vi "Get one point_test.vi"() -> ()   [LabVIEW 2017]
uses:
  <vilib>/DAQmx/read.llb/DAQmx Read (Analog DBL 1Chan 1Samp).vi
  <vilib>/DAQmx/write.llb/DAQmx Write (Analog DBL 1Chan 1Samp).vi
  <vilib>/DAQmx/create/channels.llb/DAQmx Create Channel (AO-Voltage-Basic).vi
  <vilib>/DAQmx/configure/timing.llb/DAQmx Timing (Sample Clock).vi
  <vilib>/DAQmx/create/channels.llb/DAQmx Create Channel (AI-Voltage-Basic).vi
  <vilib>/DAQmx/configure/trigger.llb/DAQmx Start Trigger (Digital Edge).vi
  <vilib>/DAQmx/configure/trigger.llb/DAQmx Start Trigger (Analog Edge).vi
  <vilib>/DAQmx/miscellaneous.llb/DAQmx Fill In Error Info.vi
panel:
  out "Time 4":dbl format="%_19f"
  out "Time 3":dbl format="%_19f"
  out "Time 2":dbl format="%_19f"
  out "Time 1":dbl format="%_19f"
  out "data":dbl format="%0.2f"
  in  "Sample Rate":dbl=500000.0 format="%.3p"
  in  "Voltage Read":tag="Dev1/ai1"
  in  "Gate":tag="Dev1/ao0"
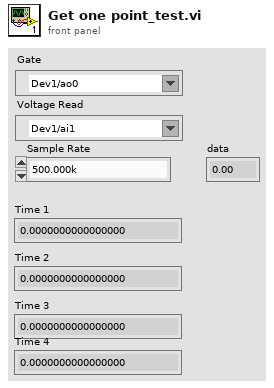
[diagram p1: front panel]
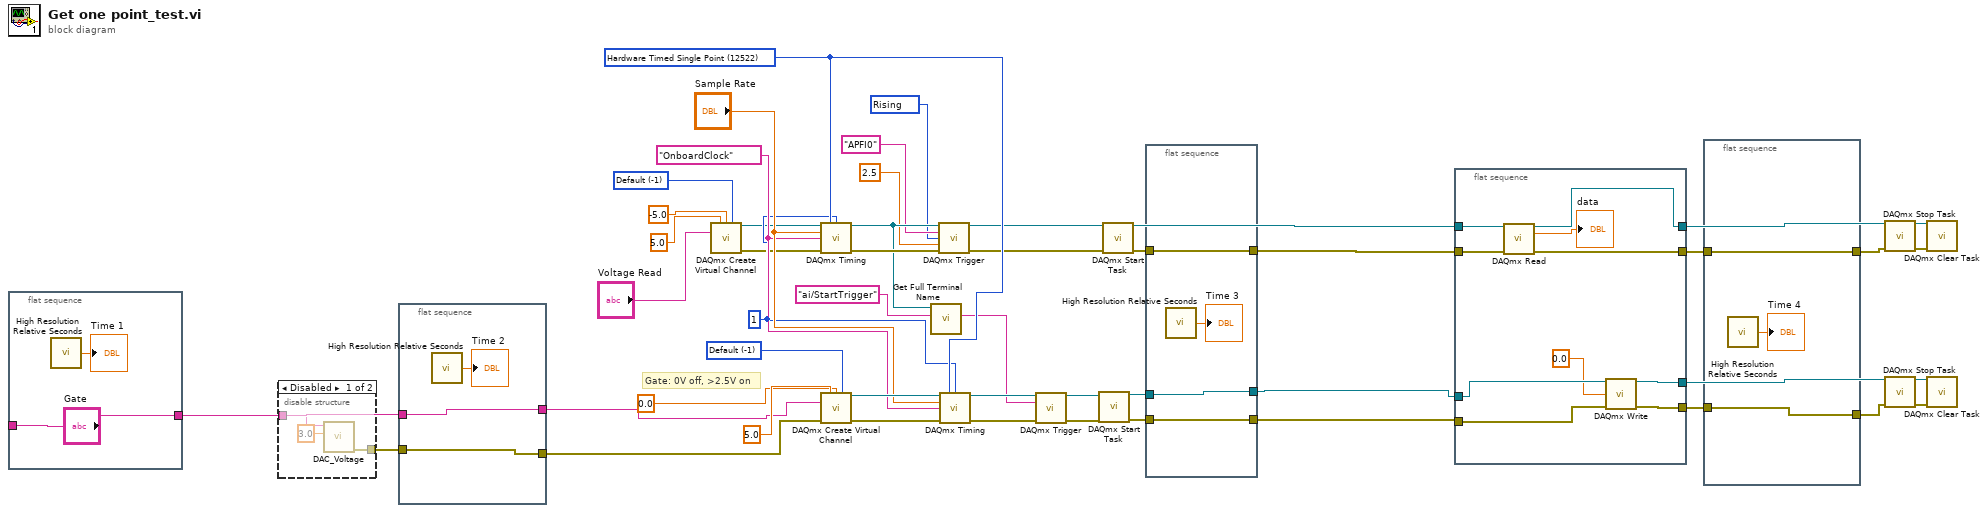
[diagram p0: block diagram]
diagram:
  w16 = 10280 items=["Rising"=10280, "Falling"=10171] ("slope")
  w36 = -1 items=["Default"=-1, "RSE"=10083, "NRSE"=10078, "Differential"=10106, "Pseudodifferential"=12529] ("input terminal configuration")
  w42 = 1 ("samples per channel")
  w43 = 12522 items=["Finite Samples"=10178, "Continuous Samples"=10123, "Hardware Timed Single Point"=12522] ("sample mode")
  w44 = tag "OnboardClock" ("source")
  w48 = -1 items=["Default"=-1, "RSE"=10083, "Differential"=10106, "Pseudodifferential"=12529] ("output terminal configuration")
  # "Gate: 0V off, >2.5V on"
  n1 = flat-sequence {
    tunnel: [w52] -> w13
    tunnel: "Gate" -> [w52]
    frame #0 {
      n2 = call <vilib>:"High Resolution Relative Seconds.vi"() -> ("relative seconds"=→"Time 1":dbl)
    }
  }
  n3 = disable-structure shown="Disabled" {
    disable-tunnel: w13 -> [w55 _]
    disable-tunnel: [w54 _] -> w11
    frame Disabled {
      n4 = call "DAC_Voltage.vi"("Voltage"=3.0, "Physical Channel(s)"=w55) -> ("error out"=w54:errorcluster)  [unwired: 9 in]
    }
    frame Enabled {
    }
  }
  n5 = flat-sequence {
    tunnel: [w58] -> w14
    tunnel: w13 -> [w58]
    tunnel: [w57] -> w12
    tunnel: w11 -> [w57]
    frame #0 {
      n6 = call <vilib>:"High Resolution Relative Seconds.vi"() -> ("relative seconds"=→"Time 2":dbl)
    }
  }
  n7 = call-poly <vilib>:"DAQmx Create Virtual Channel.vi"("maximum value"=5.0, "minimum value"=-5.0, "input terminal configuration"=w36, "physical channels"="Voltage Read") -> ("task out"=w35:refnum<k21>, "error out"=w34:errorcluster)  [unwired: 10 in]
  n8 = call-poly <vilib>:"DAQmx Timing.vi"("task/channels in"=w35, "sample mode"=w43, "samples per channel"=w42, "rate"="Sample Rate", "source"=w44, "error in"=w34) -> ("task out"=w20:refnum<k21>, "error out"=w33:errorcluster)  [unwired: 8 in]
  n9 = call-poly <vilib>:"DAQmx Create Virtual Channel.vi"("maximum value"=5.0, "minimum value"=0.0, "output terminal configuration"=w48, "physical channels"=w14, "error in"=w12) -> ("task out"=w47:refnum<k21>, "error out"=w46:errorcluster)  [unwired: 9 in]
  n10 = call "Get Full Terminal Name.vi"("Local Terminal Name"="ai/StartTrigger", "task/channels in"=w20) -> ("Terminal Name with Device Prefix"=w17:tag)  [unwired: 7 in, 2 out]
  n11 = call-poly <vilib>:"DAQmx Trigger.vi"("task/channels in"=w20, "source"="APFI0", "slope"=w16, "level"=2.5, "error in"=w33) -> ("task out"=w31:refnum<k21>, "error out"=w30:errorcluster)  [unwired: 9 in]
  n12 = call-poly <vilib>:"DAQmx Timing.vi"("task/channels in"=w47, "sample mode"=w43, "samples per channel"=w42, "rate"="Sample Rate", "source"=w44, "error in"=w46) -> ("task out"=w41:refnum<k21>, "error out"=w40:errorcluster)  [unwired: 8 in]
  n13 = call-poly <vilib>:"DAQmx Trigger.vi"("task/channels in"=w41, "source"=w17, "error in"=w40) -> ("task out"=w22:refnum<k21>, "error out"=w32:errorcluster)  [unwired: 11 in]
  n14 = call <vilib>:"DAQmx Start Task.vi"("task/channels in"=w22, "error in"=w32) -> ("task out"=w2:refnum<k21>, "error out"=w8:errorcluster)  [unwired: 12 in]
  n15 = call <vilib>:"DAQmx Start Task.vi"("task/channels in"=w31, "error in"=w30) -> ("task out"=w29:refnum<k21>, "error out"=w9:errorcluster)  [unwired: 12 in]
  n16 = flat-sequence {
    tunnel: [w62] -> w10
    tunnel: w9 -> [w62]
    tunnel: [w61] -> w1
    tunnel: w8 -> [w61]
    tunnel: [w59] -> w3
    tunnel: w2 -> [w59]
    frame #0 {
      n17 = call <vilib>:"High Resolution Relative Seconds.vi"() -> ("relative seconds"=→"Time 3":dbl)
    }
  }
  n18 = flat-sequence {
    tunnel: w3 -> [w72]
    tunnel: w29 -> [w71]
    tunnel: w10 -> [w69]
    tunnel: w1 -> [w68]
    tunnel: [w66] -> w28
    tunnel: [w65] -> w6
    tunnel: [w64] -> w23
    tunnel: [w63] -> w4
    frame #0 {
      n19 = call-poly <vilib>:"DAQmx Read.vi"("task/channels in"=w71, "error in"=w69) -> ("task out"=w64:refnum<k21>, "data"=→"data":dbl, "error out"=w63:errorcluster)  [unwired: 11 in]
      n20 = call-poly <vilib>:"DAQmx Write.vi"("task/channels in"=w72, "data"=0.0, "error in"=w68) -> ("task out"=w66:refnum<k21>, "error out"=w65:errorcluster)  [unwired: 10 in, 1 out]
    }
  }
  n21 = flat-sequence {
    tunnel: [w75] -> w7
    tunnel: w6 -> [w75]
    tunnel: [w74] -> w5
    tunnel: w4 -> [w74]
    frame #0 {
      n22 = call <vilib>:"High Resolution Relative Seconds.vi"() -> ("relative seconds"=→"Time 4":dbl)
    }
  }
  n23 = call <vilib>:"DAQmx Stop Task.vi"("task/channels in"=w23, "error in"=w5) -> ("task out"=w25:refnum<k21>, "error out"=w24:errorcluster)  [unwired: 12 in]
  n24 = call <vilib>:"DAQmx Stop Task.vi"("task/channels in"=w28, "error in"=w7) -> ("task out"=w27:refnum<k21>, "error out"=w26:errorcluster)  [unwired: 12 in]
  n25 = call <vilib>:"DAQmx Clear Task.vi"("task in"=w25, "error in"=w24) -> ()  [unwired: 13 in, 1 out]
  n26 = call <vilib>:"DAQmx Clear Task.vi"("task in"=w27, "error in"=w26) -> ()  [unwired: 13 in, 1 out]
